vi "Zeiss File Header Tclk.vi"(7 "Write":bool=TRUE, 8 "error in":errorcluster, 9 "Inputs":T2={"AI sampling time increment"=0.0, "8-bit"=TRUE, "AI scaling coefficients"=[], "AI channels"={"AI 1"=FALSE, "AI 2"=FALSE, "AI 3"=FALSE, "AI 4"=FALSE}, "Resolution and scan"={"X resolution"=1, "Z resolution"=1, "AI oversampling"=1, "Scan speed"=1, "Actual AO rate"=1.0, "Frame line rampdown ratio"=1.0, "X min (V)"=0.0, "X max (V)"=0.0, "Det min (V)"=-10.0, "Det max (V)"=10.0}, "Decimating factor"=2, "Notes"="", "Other detectors"={"Detector C name"="", "Detector D name"=""}, "SEM parameters"={"Detector A"="", "Detector B"="Detecter B name", "Brightness A"=0.0, "Contrast A"=0.0, "Brightness B"=0.0, "Contrast B"=0.0, "Magnification"=0.0, "Pixel size"=0.0, "Working distance"=0.0, "EHT"=0.0, "Aperture"=0, "High current mode"=0, "Probe current"=0.0, "Scan rotation"=0.0, "Chamber vac"=0.0, "Gun vac"=0.0, "Beam shift X"=0.0, "Beam shift Y"=0.0, "Stig X"=0.0, "Stig Y"=0.0, "Alignment X"=0.0, "Alignment Y"=0.0, "Stage X"=0.0, "Stage Y"=0.0, "Stage Z"=0.0, "Stage T"=0.0, "Stage R"=0.0, "Stage M"=0.0}, "FIB parameters"={"FIB mode"=0, "FIB focus"=0.0, "FIB probe current"=0, "FIB emission current"=0.0, "FIB rotation"=0.0, "FIB aperture X"=0.0, "FIB aperture Y"=0.0, "FIB stig X"=0.0, "FIB stig Y"=0.0, "FIB beam shift X"=0.0, "FIB beam shift Y"=0.0}, "Milling para"={"X resolution"=4096, "Z resolution"=125001, "X offset (um)"=0.0, "Z offset (um)"=0.0, "X center (um)"=0.0, "Z center (um)"=0.0, "X size (um)"=250.0, "Z size (um)"=250.0, "UL-Ang"=90.0, "UR-Ang"=90.0, "Line milling time (s)"=5.0, "Z-step (nm)"=2.0, "Lines auto pause"=1, "Auto pause"=FALSE, "Mill from Bottom"=FALSE, "FIB FOV (um)"=500.0, "Auto Profile"=FALSE, "Mill start from Last"=FALSE, "FIB PID on"=FALSE, "FIB PID reset"=TRUE, "FIB PID measured"=0, "FIB PID target"=0.0, "FIB PID target slope"=0.0, "FIB PID P"=0.001, "FIB PID I"=0.01, "FIB PID D"=0.0, "Emission (uA)"=1.36, "Suppressor (V)"=50.0, "Auto reheat"=FALSE}, "Machine ID"="", "Data Logging"={"Temp (F)"=0.0, "FIB Faraday Cup (nA)"=0.0, "FIB Specimen I (nA)"=0.0, "Beam Dump 1 (nA)"=0.0, "Beam Dump 2 (nA)"=0.0, "Milling I (nA)"=0.0, "SEM Specimen I (nA)"=0.0, "Milling Z voltage (V)"=0.0, "Focus Index"=0.0, "FIB slice #"=0}} {"Milling para"."Suppressor (V)" step=0.1 format="%.1g"; "Milling para"."Emission (uA)" step=0.1 format="%.2g"; "Milling para"."FIB PID measured" items=["Spec.", "B.D. 1", "B.D. 2", "Mill", "Spec. +"]; "Milling para"."FIB PID target slope" min=-1 max=1 step=0.1; "Milling para"."UR-Ang" format="%.2f"; "Milling para"."UL-Ang" format="%.2f"; "Milling para"."Z offset (um)" step=0.02 format="%.3g"; "Milling para"."X offset (um)" step=1 format="%.3g"; "Milling para"."FIB FOV (um)" format="%.3g"; "Milling para"."Line milling time (s)" format="%.1f"; "Milling para"."Z center (um)" format="%#.3g"; "Milling para"."X center (um)" format="%#.3g"; "Data Logging"."Milling I (nA)" format="%.2g"; "Data Logging"."Beam Dump 2 (nA)" format="%.2g"; "Data Logging"."Focus Index" format="%#_3g"; "Data Logging"."Milling Z voltage (V)" format="%.4g"; "Data Logging"."SEM Specimen I (nA)" format="%.2g"; "Data Logging"."Beam Dump 1 (nA)" format="%.2g"; "Data Logging"."FIB Specimen I (nA)" format="%.2g"; "Data Logging"."FIB Faraday Cup (nA)" format="%.2g"; "Data Logging"."Temp (F)" format="%.2g"}, 10 "Input file path":path, 11 "refnum":refnum<file>) -> (0 "error out":errorcluster, 1 "Ouputs":T1={"AI sampling time increment"=0.0, "AI scaling coefficients"=[], "AI channels"={"AI 1"=FALSE, "AI 2"=FALSE, "AI 3"=FALSE, "AI 4"=FALSE}, "Resolution and scan"={"X resolution"=1, "Z resolution"=1, "AI oversampling"=1, "Scan speed"=1, "Actual AO rate"=1.0, "Frame line rampdown ratio"=1.0, "X min (V)"=0.0, "X max (V)"=0.0, "Det min (V)"=-10.0, "Det max (V)"=10.0}, "Decimating factor"=2, "Notes"="", "Other detectors"={"Detector C name"="", "Detector D name"=""}, "SEM parameters"={"Detector A"="", "Detector B"="Detecter B name", "Brightness A"=0.0, "Contrast A"=0.0, "Brightness B"=0.0, "Contrast B"=0.0, "Magnification"=0.0, "Pixel size"=0.0, "Working distance"=0.0, "EHT"=0.0, "Aperture"=0, "High current mode"=0, "Probe current"=0.0, "Scan rotation"=0.0, "Chamber vac"=0.0, "Gun vac"=0.0, "Beam shift X"=0.0, "Beam shift Y"=0.0, "Stig X"=0.0, "Stig Y"=0.0, "Alignment X"=0.0, "Alignment Y"=0.0, "Stage X"=0.0, "Stage Y"=0.0, "Stage Z"=0.0, "Stage T"=0.0, "Stage R"=0.0, "Stage M"=0.0}, "FIB parameters"={"FIB mode"=0, "FIB focus"=0.0, "FIB probe current"=0, "FIB emission current"=0.0, "FIB rotation"=0.0, "FIB aperture X"=0.0, "FIB aperture Y"=0.0, "FIB stig X"=0.0, "FIB stig Y"=0.0, "FIB beam shift X"=0.0, "FIB beam shift Y"=0.0}, "Milling para"={"X resolution"=4096, "Z resolution"=125001, "X offset (um)"=0.0, "Z offset (um)"=0.0, "X center (um)"=0.0, "Z center (um)"=0.0, "X size (um)"=250.0, "Z size (um)"=250.0, "UL-Ang"=90.0, "UR-Ang"=90.0, "Line milling time (s)"=5.0, "Z-step (nm)"=2.0, "Lines auto pause"=1, "Auto pause"=FALSE, "Mill from Bottom"=FALSE, "FIB FOV (um)"=500.0, "Auto Profile"=FALSE, "Mill start from Last"=FALSE, "FIB PID on"=FALSE, "FIB PID reset"=TRUE, "FIB PID measured"=0, "FIB PID target"=0.0, "FIB PID target slope"=0.0, "FIB PID P"=0.001, "FIB PID I"=0.01, "FIB PID D"=0.0, "Emission (uA)"=1.36, "Suppressor (V)"=50.0, "Auto reheat"=FALSE}, "Machine ID"="", "Data Logging"={"Temp (F)"=0.0, "FIB Faraday Cup (nA)"=0.0, "FIB Specimen I (nA)"=0.0, "Beam Dump 1 (nA)"=0.0, "Beam Dump 2 (nA)"=0.0, "Milling I (nA)"=0.0, "SEM Specimen I (nA)"=0.0, "Milling Z voltage (V)"=0.0, "Focus Index"=0.0, "FIB slice #"=0}} {"Milling para"."Suppressor (V)" step=0.1 format="%.1g"; "Milling para"."Emission (uA)" step=0.1 format="%.2g"; "Milling para"."FIB PID measured" items=["Spec.", "B.D. 1", "B.D. 2", "Mill", "Spec. +"]; "Milling para"."FIB PID target slope" min=-1 max=1 step=0.1; "Milling para"."UR-Ang" format="%.2f"; "Milling para"."UL-Ang" format="%.2f"; "Milling para"."Z offset (um)" step=0.02 format="%.3g"; "Milling para"."X offset (um)" step=1 format="%.3g"; "Milling para"."FIB FOV (um)" format="%.3g"; "Milling para"."Line milling time (s)" format="%.1f"; "Milling para"."Z center (um)" format="%#.3g"; "Milling para"."X center (um)" format="%#.3g"; "Data Logging"."Milling I (nA)" format="%.2g"; "Data Logging"."Beam Dump 2 (nA)" format="%.2g"; "Data Logging"."Focus Index" format="%#_3g"; "Data Logging"."Milling Z voltage (V)" format="%.4g"; "Data Logging"."SEM Specimen I (nA)" format="%.2g"; "Data Logging"."Beam Dump 1 (nA)" format="%.2g"; "Data Logging"."FIB Specimen I (nA)" format="%.2g"; "Data Logging"."FIB Faraday Cup (nA)" format="%.2g"; "Data Logging"."Temp (F)" format="%.2g"}, 3 "dup refnum":refnum<file>)   [LabVIEW 2018]
panel:
  in  "Detector calibration":sgl[](array[numeric])=[0.0, 0.0, 0.0, 0.0]
  out "SW date":string
  out "Detectors":refnum<k15>="PXI1Slot3"
  # "Direction"
  # "Start\nfrom"
  # "<"
  # "Direction"
  # "Start\nfrom"
  # "<"
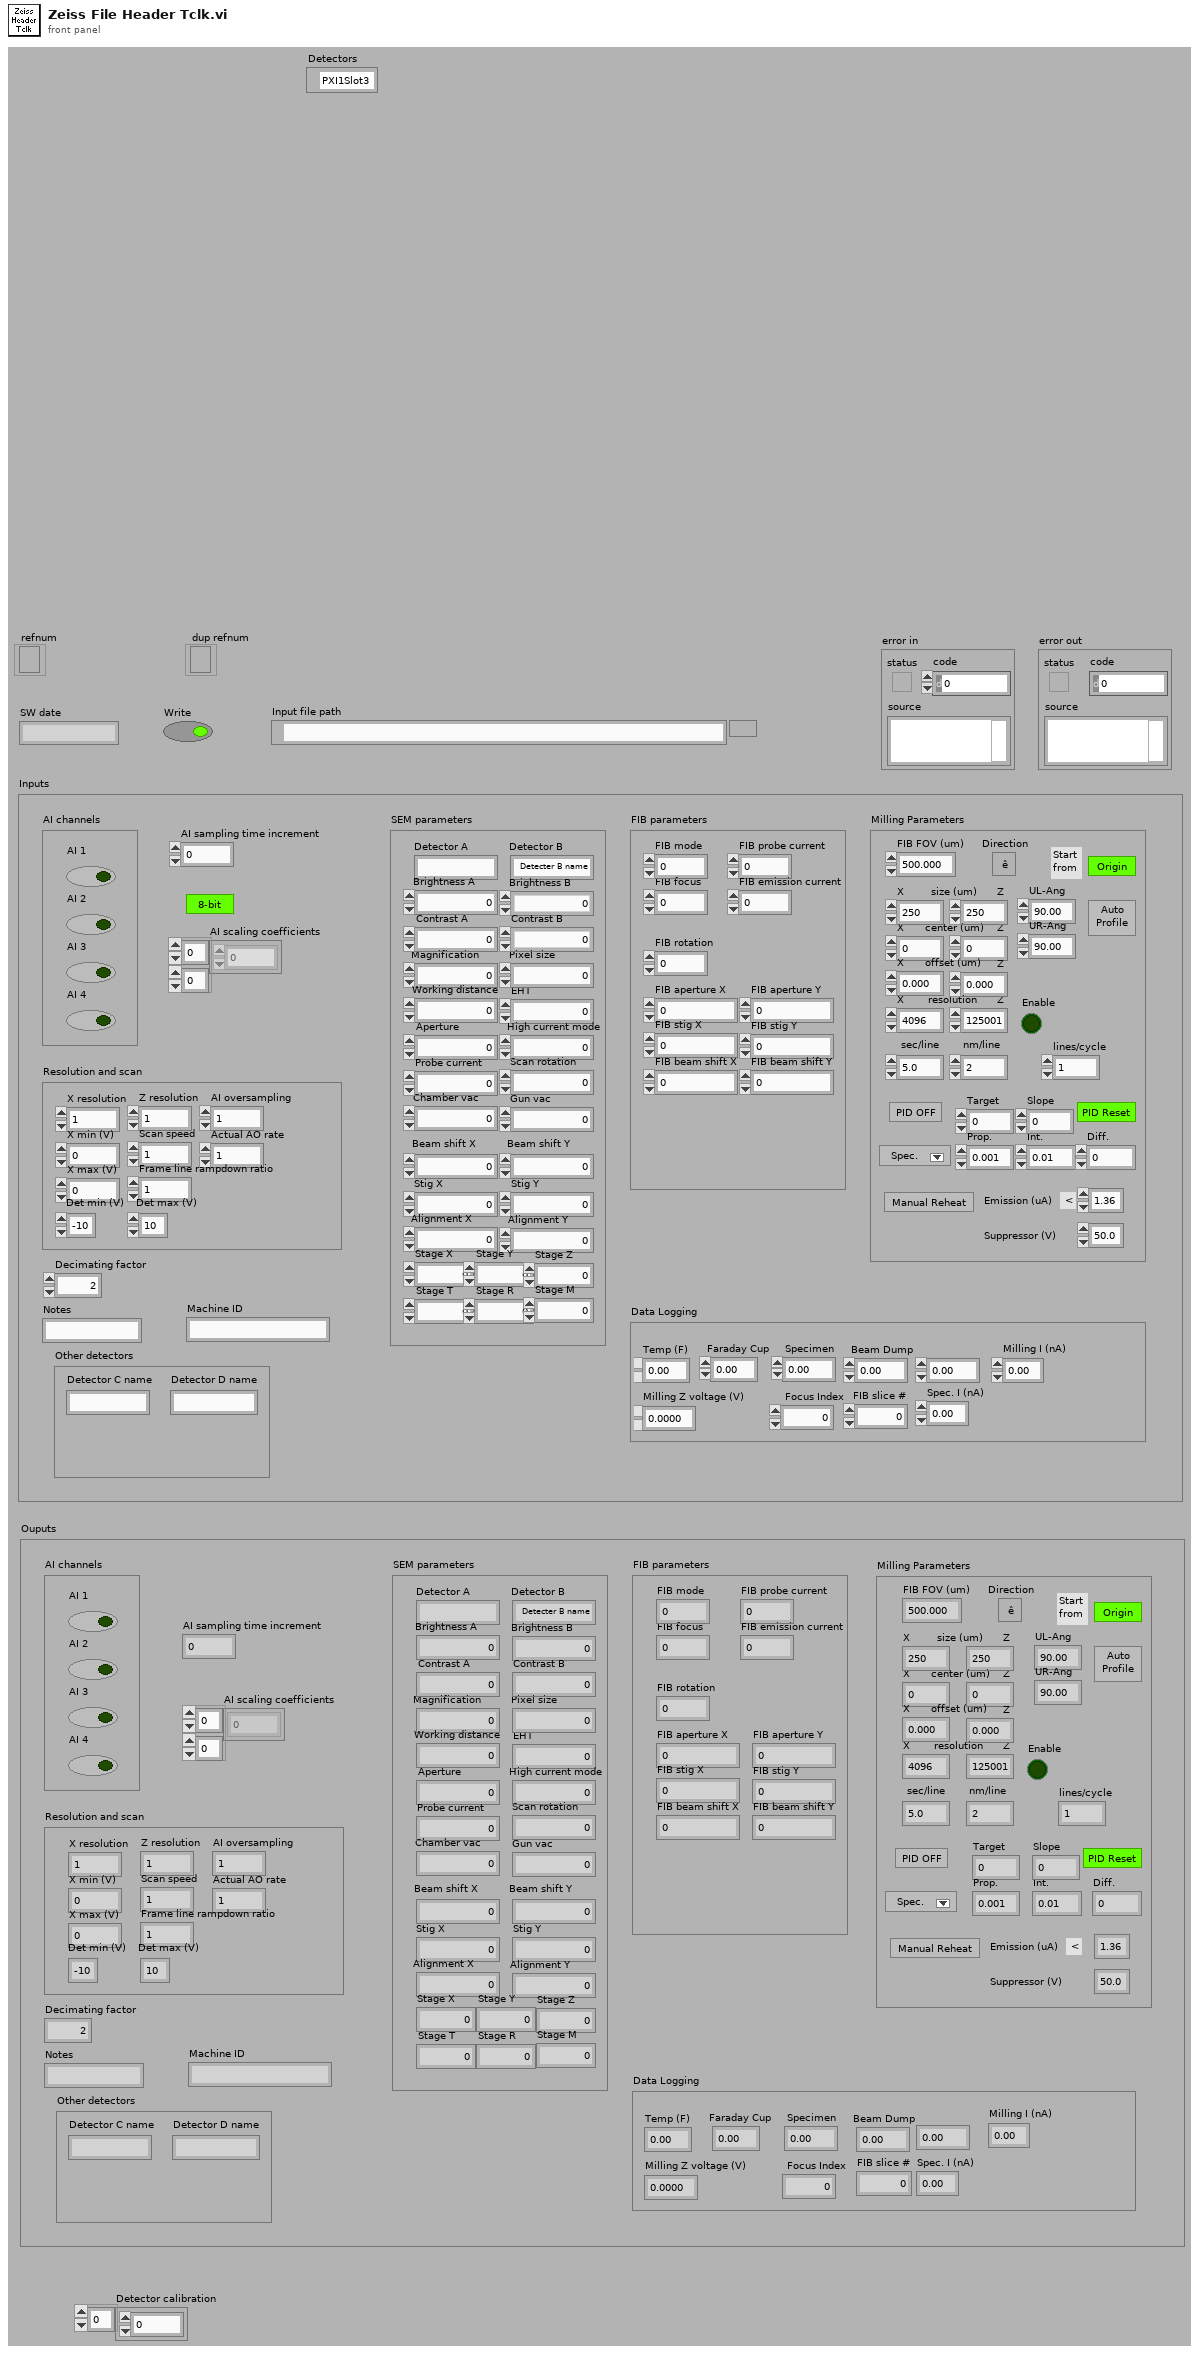
[diagram p1: front panel]
types:
  T1 = cluster{"AI sampling time increment":dbl, "AI scaling coefficients":sgl[][], "AI channels":cluster{"AI 1":bool, "AI 2":bool, "AI 3":bool, "AI 4":bool}, "Resolution and scan":cluster{"X resolution":u32, "Z resolution":u32, "AI oversampling":u16, "Scan speed":u8, "Actual AO rate":dbl, "Frame line rampdown ratio":dbl, "X min (V)":dbl, "X max (V)":dbl, "Det min (V)":dbl, "Det max (V)":dbl}, "Decimating factor":u16, "Notes":string, "Other detectors":cluster{"Detector C name":string, "Detector D name":string}, "SEM parameters":cluster{"Detector A":string, "Detector B":string, "Brightness A":sgl, "Contrast A":sgl, "Brightness B":sgl, "Contrast B":sgl, "Magnification":sgl, "Pixel size":sgl, "Working distance":sgl, "EHT":sgl, "Aperture":u8, "High current mode":u8, "Probe current":sgl, "Scan rotation":sgl, "Chamber vac":sgl, "Gun vac":sgl, "Beam shift X":sgl, "Beam shift Y":sgl, "Stig X":sgl, "Stig Y":sgl, "Alignment X":sgl, "Alignment Y":sgl, "Stage X":sgl, "Stage Y":sgl, "Stage Z":sgl, "Stage T":sgl, "Stage R":sgl, "Stage M":sgl}, "FIB parameters":cluster{"FIB mode":u8, "FIB focus":sgl, "FIB probe current":u8, "FIB emission current":sgl, "FIB rotation":sgl, "FIB aperture X":sgl, "FIB aperture Y":sgl, "FIB stig X":sgl, "FIB stig Y":sgl, "FIB beam shift X":sgl, "FIB beam shift Y":sgl}, "Milling para":cluster{"X resolution":u32, "Z resolution":u32, "X offset (um)":sgl, "Z offset (um)":sgl, "X center (um)":sgl, "Z center (um)":sgl, "X size (um)":sgl, "Z size (um)":sgl, "UL-Ang":sgl, "UR-Ang":sgl, "Line milling time (s)":sgl, "Z-step (nm)":dbl, "Lines auto pause":u16, "Auto pause":bool, "Mill from Bottom":bool, "FIB FOV (um)":sgl, "Auto Profile":bool, "Mill start from Last":bool, "FIB PID on":bool, "FIB PID reset":bool, "FIB PID measured":u8, "FIB PID target":sgl, "FIB PID target slope":sgl, "FIB PID P":sgl, "FIB PID I":sgl, "FIB PID D":sgl, "Emission (uA)":dbl, "Suppressor (V)":sgl, "Auto reheat":bool}, "Machine ID":string, "Data Logging":cluster{"Temp (F)":sgl, "FIB Faraday Cup (nA)":sgl, "FIB Specimen I (nA)":sgl, "Beam Dump 1 (nA)":sgl, "Beam Dump 2 (nA)":sgl, "Milling I (nA)":sgl, "SEM Specimen I (nA)":sgl, "Milling Z voltage (V)":sgl, "Focus Index":sgl, "FIB slice #":u32}}
  T2 = cluster{"AI sampling time increment":dbl, "8-bit":bool, "AI scaling coefficients":sgl[][], "AI channels":cluster{"AI 1":bool, "AI 2":bool, "AI 3":bool, "AI 4":bool}, "Resolution and scan":cluster{"X resolution":u32, "Z resolution":u32, "AI oversampling":u16, "Scan speed":u8, "Actual AO rate":dbl, "Frame line rampdown ratio":dbl, "X min (V)":dbl, "X max (V)":dbl, "Det min (V)":dbl, "Det max (V)":dbl}, "Decimating factor":u16, "Notes":string, "Other detectors":cluster{"Detector C name":string, "Detector D name":string}, "SEM parameters":cluster{"Detector A":string, "Detector B":string, "Brightness A":sgl, "Contrast A":sgl, "Brightness B":sgl, "Contrast B":sgl, "Magnification":sgl, "Pixel size":sgl, "Working distance":sgl, "EHT":sgl, "Aperture":u8, "High current mode":u8, "Probe current":sgl, "Scan rotation":sgl, "Chamber vac":sgl, "Gun vac":sgl, "Beam shift X":sgl, "Beam shift Y":sgl, "Stig X":sgl, "Stig Y":sgl, "Alignment X":sgl, "Alignment Y":sgl, "Stage X":sgl, "Stage Y":sgl, "Stage Z":sgl, "Stage T":sgl, "Stage R":sgl, "Stage M":sgl}, "FIB parameters":cluster{"FIB mode":u8, "FIB focus":sgl, "FIB probe current":u8, "FIB emission current":sgl, "FIB rotation":sgl, "FIB aperture X":sgl, "FIB aperture Y":sgl, "FIB stig X":sgl, "FIB stig Y":sgl, "FIB beam shift X":sgl, "FIB beam shift Y":sgl}, "Milling para":cluster{"X resolution":u32, "Z resolution":u32, "X offset (um)":sgl, "Z offset (um)":sgl, "X center (um)":sgl, "Z center (um)":sgl, "X size (um)":sgl, "Z size (um)":sgl, "UL-Ang":sgl, "UR-Ang":sgl, "Line milling time (s)":sgl, "Z-step (nm)":dbl, "Lines auto pause":u16, "Auto pause":bool, "Mill from Bottom":bool, "FIB FOV (um)":sgl, "Auto Profile":bool, "Mill start from Last":bool, "FIB PID on":bool, "FIB PID reset":bool, "FIB PID measured":u8, "FIB PID target":sgl, "FIB PID target slope":sgl, "FIB PID P":sgl, "FIB PID I":sgl, "FIB PID D":sgl, "Emission (uA)":dbl, "Suppressor (V)":sgl, "Auto reheat":bool}, "Machine ID":string, "Data Logging":cluster{"Temp (F)":sgl, "FIB Faraday Cup (nA)":sgl, "FIB Specimen I (nA)":sgl, "Beam Dump 1 (nA)":sgl, "Beam Dump 2 (nA)":sgl, "Milling I (nA)":sgl, "SEM Specimen I (nA)":sgl, "Milling Z voltage (V)":sgl, "Focus Index":sgl, "FIB slice #":u32}}
  T3 = cluster{"Detector C name":string, "Detector D name":string}
  T4 = cluster{"FIB mode":u8, "FIB focus":sgl, "FIB probe current":u8, "FIB emission current":sgl, "FIB rotation":sgl, "FIB aperture X":sgl, "FIB aperture Y":sgl, "FIB stig X":sgl, "FIB stig Y":sgl, "FIB beam shift X":sgl, "FIB beam shift Y":sgl}
  T5 = cluster{"Temp (F)":sgl, "FIB Faraday Cup (nA)":sgl, "FIB Specimen I (nA)":sgl, "Beam Dump 1 (nA)":sgl, "Beam Dump 2 (nA)":sgl, "Milling I (nA)":sgl, "SEM Specimen I (nA)":sgl, "Milling Z voltage (V)":sgl, "Focus Index":sgl, "FIB slice #":u32}
  T6 = cluster{"Detector A":string, "Detector B":string, "Brightness A":sgl, "Contrast A":sgl, "Brightness B":sgl, "Contrast B":sgl, "Magnification":sgl, "Pixel size":sgl, "Working distance":sgl, "EHT":sgl, "Aperture":u8, "High current mode":u8, "Probe current":sgl, "Scan rotation":sgl, "Chamber vac":sgl, "Gun vac":sgl, "Beam shift X":sgl, "Beam shift Y":sgl, "Stig X":sgl, "Stig Y":sgl, "Alignment X":sgl, "Alignment Y":sgl, "Stage X":sgl, "Stage Y":sgl, "Stage Z":sgl, "Stage T":sgl, "Stage R":sgl, "Stage M":sgl}
  T7 = cluster{"AI 1":bool, "AI 2":bool, "AI 3":bool, "AI 4":bool}
  T8 = cluster{"X resolution":u32, "Z resolution":u32, "AI oversampling":u16, "Scan speed":u8, "Actual AO rate":dbl, "Frame line rampdown ratio":dbl, "X min (V)":dbl, "X max (V)":dbl, "Det min (V)":dbl, "Det max (V)":dbl}
  T9 = cluster{"X resolution":u32, "Z resolution":u32, "X offset (um)":sgl, "Z offset (um)":sgl, "X center (um)":sgl, "Z center (um)":sgl, "X size (um)":sgl, "Z size (um)":sgl, "UL-Ang":sgl, "UR-Ang":sgl, "Line milling time (s)":sgl, "Z-step (nm)":dbl, "Lines auto pause":u16, "Auto pause":bool, "Mill from Bottom":bool, "FIB FOV (um)":sgl, "Auto Profile":bool, "Mill start from Last":bool, "FIB PID on":bool, "FIB PID reset":bool, "FIB PID measured":u8, "FIB PID target":sgl, "FIB PID target slope":sgl, "FIB PID P":sgl, "FIB PID I":sgl, "FIB PID D":sgl, "Emission (uA)":dbl, "Suppressor (V)":sgl, "Auto reheat":bool}
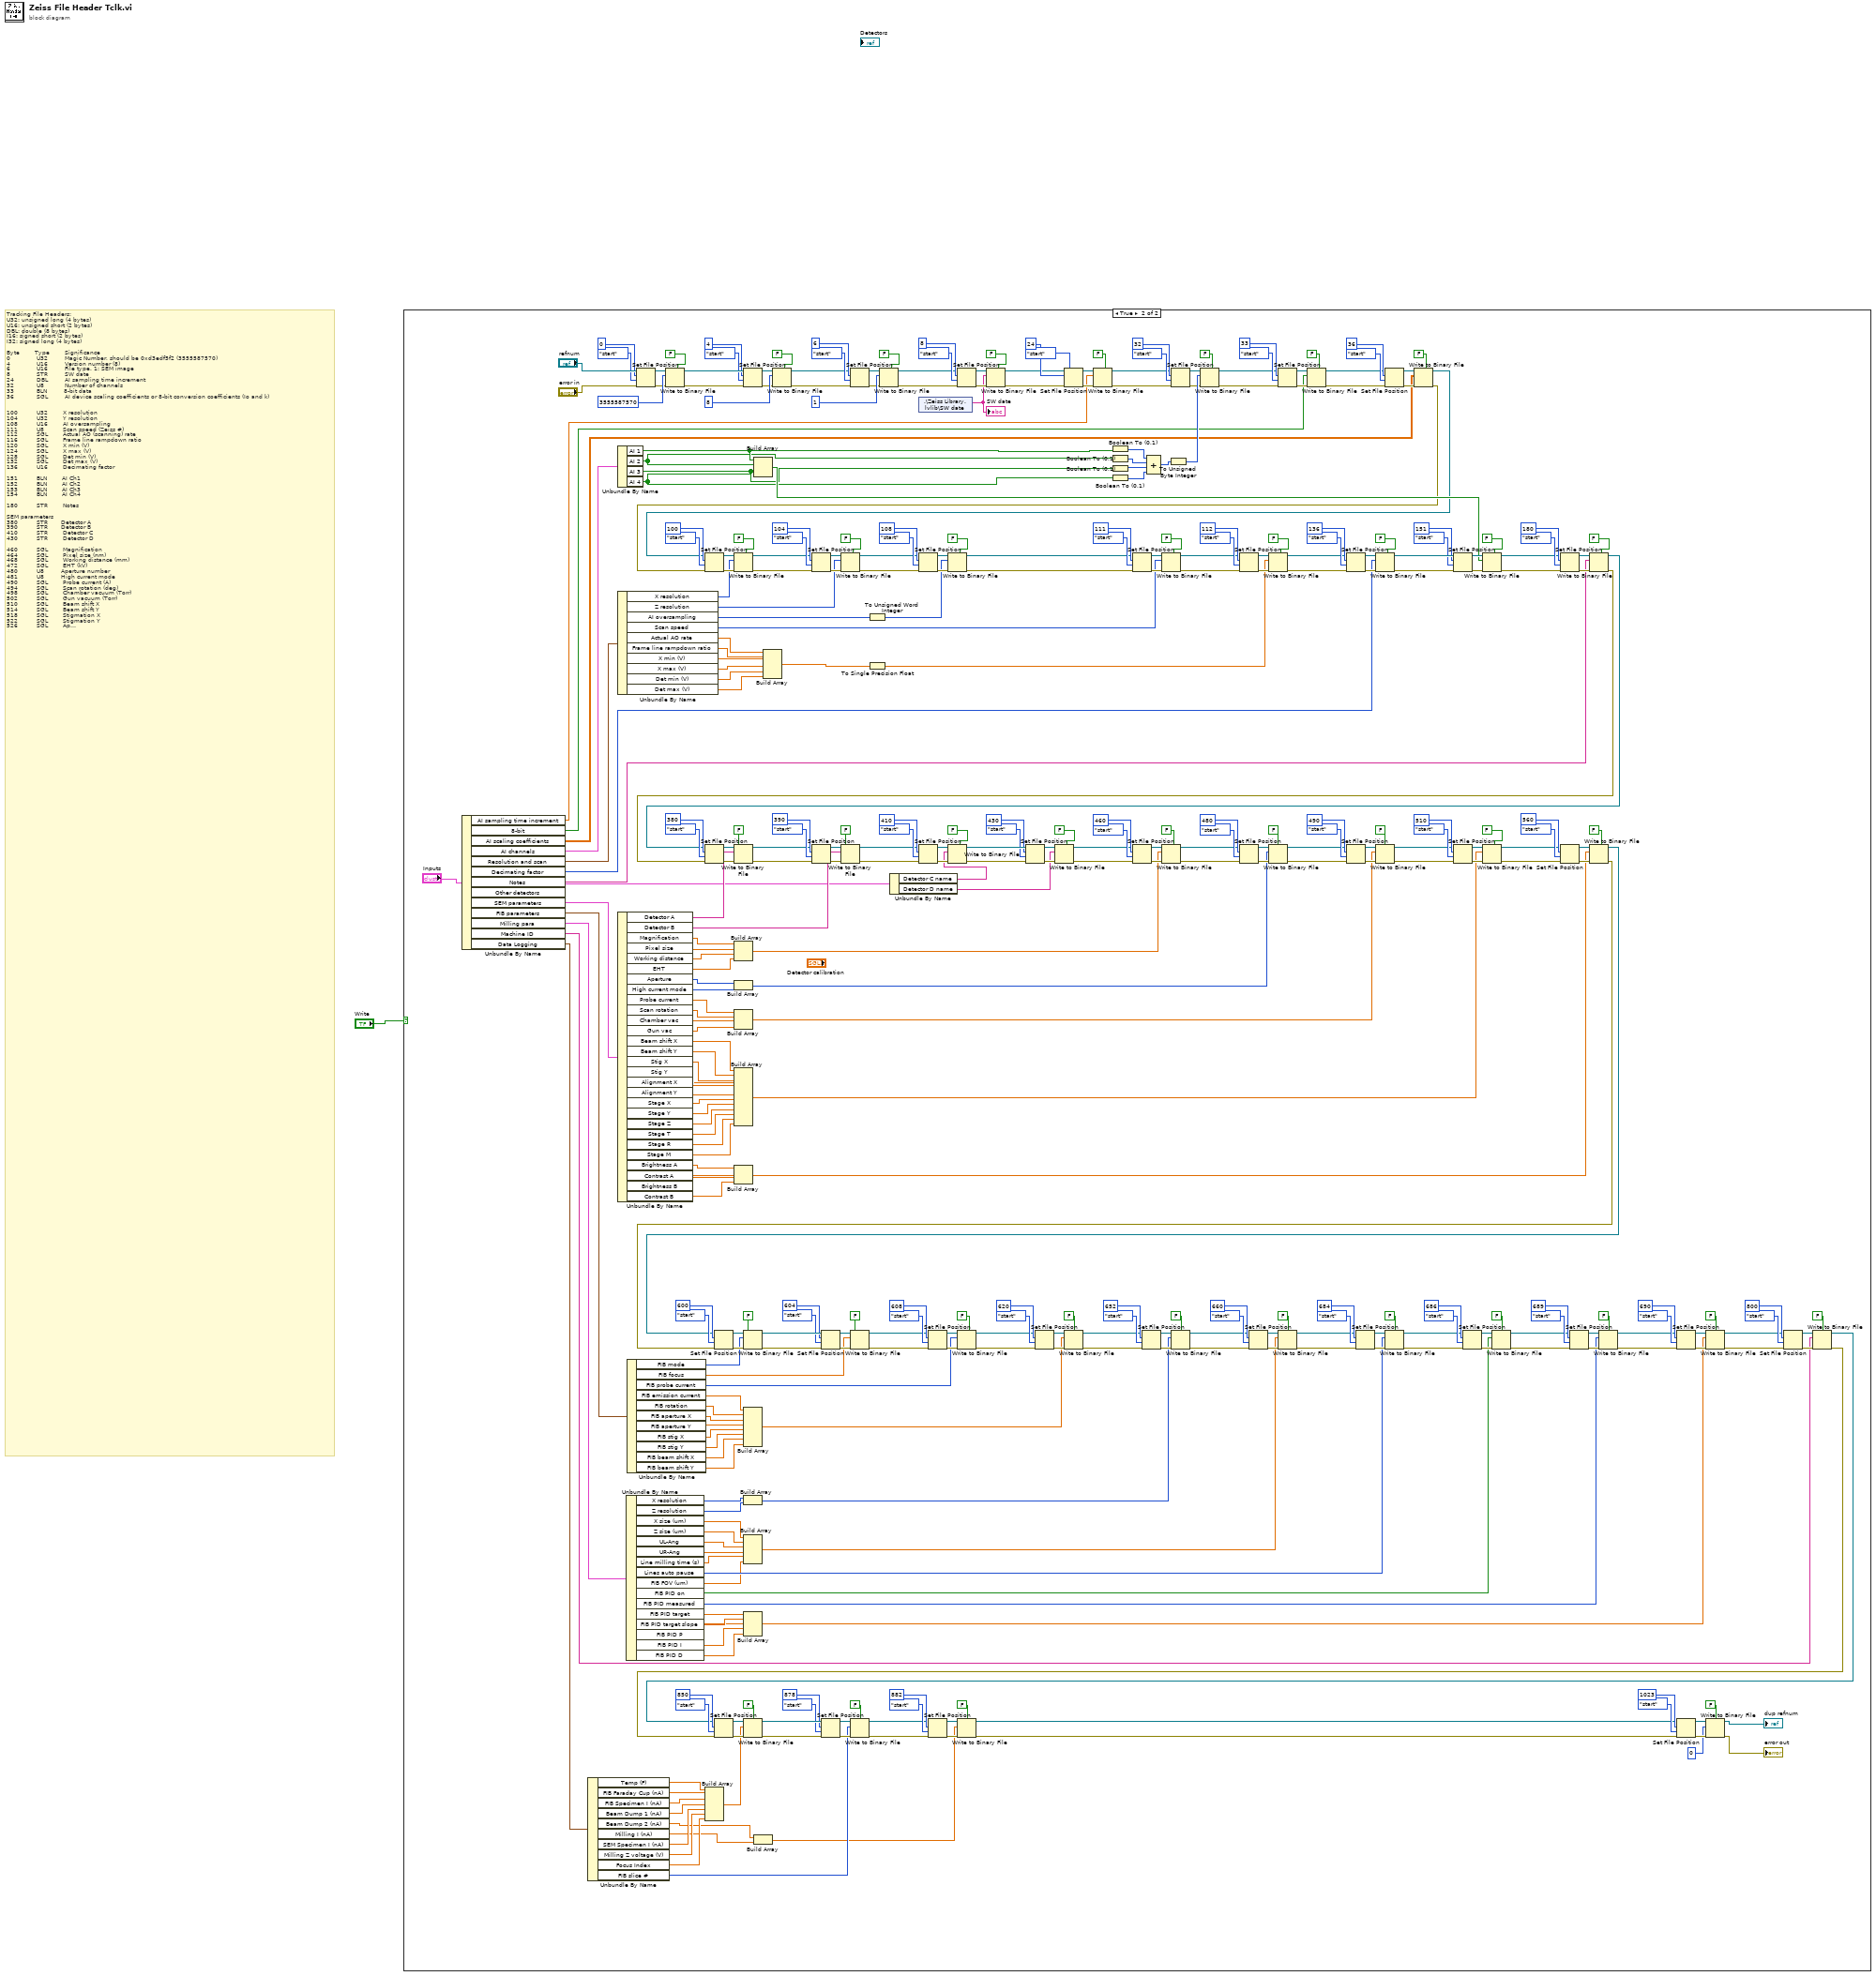
[diagram p0: block diagram]
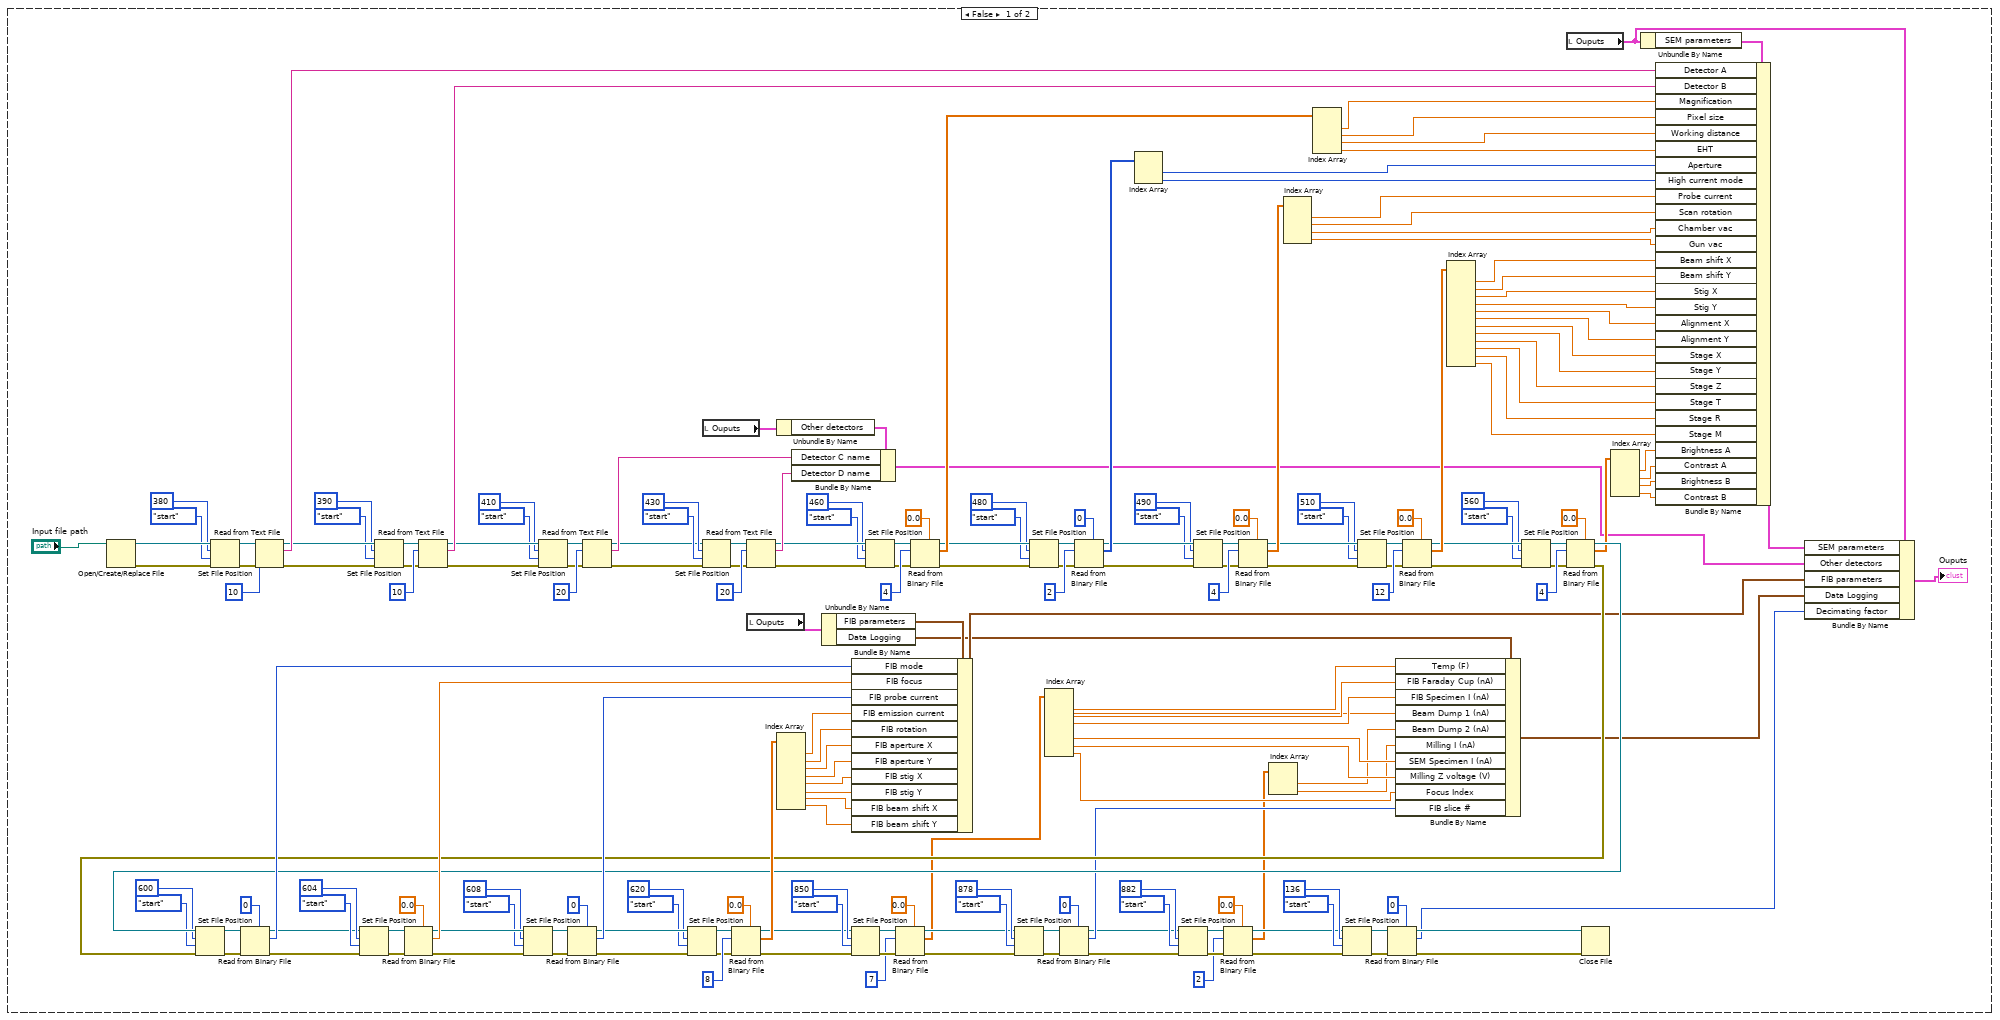
[diagram p2: hidden frame]
diagram:
  # "Tracking File Headers:\nU32: unsigned long (4 bytes)\nU16: unsigned short (2 bytes)\nDBL: double (8 bytes)\nI16: signed short (2 bytes)\nI32: signed long (4 bytes)\n\nByte\t       Type\t\t      Significance\n0              U32\t        Magic Number, should be 0xd3edf5f2 (3555587570)\n4   \t          U16\t        Version number (8)\n6   \t          U16\t        File type. 1: SEM image\n8              STR         SW date\n24     \t      DBL         AI sampling time increment\n32     \t      U8           Number of channels\n33            BLN         8-bit data\n36            SGL         AI device scaling coefficients or 8-bit conversion coefficients (Io and k)\n\n\n100          U32        X resolution\n104          U32        Y resolution\n108          U16        AI oversampling     \n111          U8          Scan speed (Zeiss #)\n112          SGL        Actual AO (scanning) rate\n116          SGL        Frame line rampdown ratio\n120          SGL        X min (V)\n124          SGL        X max (V)\n128          SGL        Det min (V)\n132          SGL        Det max (V)\n136          U16        Decimating factor \n\n151          BLN        AI Ch1          \n152          BLN        AI Ch2\n153          BLN        AI Ch3\n154          BLN        AI Ch4\n \n180          STR        Notes\n\nSEM parameters\n380          STR       Detector A\n390          STR       Detector B\n410          STR        Detector C\n430          STR        Detector D\n\n460          SGL        Magnification\n464          SGL        Pixel size (nm)\n468          SGL        Working distance (mm)\n472          SGL        EHT (kV)\n480          U8         Aperture number\n481          U8         High current mode\n490          SGL        Probe current (A)\n494          SGL        Scan rotation (deg)\n498          SGL        Chamber vacuum (Torr)\n502          SGL        Gun vacuum (Torr)\n510          SGL        Beam shift X\n514          SGL        Beam shift Y\n518          SGL        Stigmation X\n522          SGL        Stigmation Y\n526          SGL        Aperture aligment X\n530          SGL        Aperture aligment Y\n534          SGL        Stage X (mm)\n538          SGL        Stage Y (mm)\n542          SGL        Stage Z (mm)\n546          SGL        Stage T (deg)\n550          SGL        Stage R (deg)\n554          SGL        Stage M (mm)\n560          SGL        Brightness (%), detector A\n564          SGL        Contrast (%),  detector A\n568          SGL        Brightness (%), detector B\n572          SGL        Contrast (%),  detector B\n\n\nFIB parameters\n600          U8         Mode\n604          SGL        Focus (V)\n608          U8         Probe current number\n620          SGL        Emission current (A)\n624          SGL        rotation (deg)\n628          SGL        Aperture alignment X\n632          SGL        Aperture alignment Y\n636          SGL        Stigmation X\n640          SGL        Stigmation Y\n644          SGL        Beam shift X (um)\n648          SGL        Beam shift Y (um)\n\n\nMilling parameters\n652          U32        X resolution\n656          U32        Y resolution\n660          SGL        X size (um)\n664          SGL        Y size (um)\n668          SGL        UL-Ang (deg)\n672          SGL        UR-Ang (deg)\n676          SGL        Line milling time (s)\n680          SGL        FIB FOV (um)\n684          U16        Lines auto pause\n686          BLN       FIB PID on\n689          U8          FIB PID measured (0: specimen, 1: beam dump)\n690          SGL        FIB PID target\n694          SGL        FIB PID target slope\n698          SGL        FIB PID P\n702          SGL        FIB PID I\n706          SGL        FIB PID D\n\n\n800          STR        Machine ID\n\n850          SGL        Temperature (F)\n854          SGL        Faraday cup current (nA)\n858          SGL        Specimen current during FIB (nA)\n862          SGL        Beam dump 1 current (nA)\n866          SGL        Specimen current during SEM (nA)\n870          SGL        Milling Z voltage (V)\n874          SGL        Focus index\n878          U32        FIB slice #\n882          SGL        Beam dump 2 current (nA)\n886          SGL        Milling current (nA)\n\n1000        DBL        File length, position for the beginning of recipe variant\n\n1024        I16          1-D array of n channels of unscaled measurement from DAQ"
  n1 = case shown="True" "Write" {
    frame False {
      n2 = Open/Create/Replace File(file path (use dialog)="Input file path") -> (refnum out=w111:refnum<file>, error out=w112:errorcluster)  [unwired: 5 in, 1 out]
      n3 = Set File Position(offset (in bytes) (0)=380 ("pos offset (0)"), refnum=w111, from (0:start)=enum16{"start", "end", "current"}."start" ("pos mode (0:2)"), error in=w112) -> (refnum out=w81:refnum<file>, error out=w82:errorcluster)
      n4 = Read from Text File(file (use dialog)=w81, count=10, error in=w82) -> (refnum out=w91:refnum<file>, text=w121:string, error out=w92:errorcluster)  [unwired: 1 in, 1 out]
      n5 = Set File Position(offset (in bytes) (0)=390 ("pos offset (0)"), refnum=w91, from (0:start)=enum16{"start", "end", "current"}."start" ("pos mode (0:2)"), error in=w92) -> (refnum out=w89:refnum<file>, error out=w90:errorcluster)
      n6 = Read from Text File(file (use dialog)=w89, count=10, error in=w90) -> (refnum out=w103:refnum<file>, text=w122:string, error out=w104:errorcluster)  [unwired: 1 in, 1 out]
      n7 = Set File Position(offset (in bytes) (0)=410 ("pos offset (0)"), refnum=w103, from (0:start)=enum16{"start", "end", "current"}."start" ("pos mode (0:2)"), error in=w104) -> (refnum out=w96:refnum<file>, error out=w95:errorcluster)
      n8 = Read from Text File(file (use dialog)=w96, count=20, error in=w95) -> (refnum out=w94:refnum<file>, text=w119:string, error out=w93:errorcluster)  [unwired: 1 in, 1 out]
      n9 = local read "Ouputs"() -> (w57:T1)
      n10 = Set File Position(offset (in bytes) (0)=430 ("pos offset (0)"), refnum=w94, from (0:start)=enum16{"start", "end", "current"}."start" ("pos mode (0:2)"), error in=w93) -> (refnum out=w101:refnum<file>, error out=w102:errorcluster)
      n11 = Read from Text File(file (use dialog)=w101, count=20, error in=w102) -> (refnum out=w105:refnum<file>, text=w120:string, error out=w106:errorcluster)  [unwired: 1 in, 1 out]
      n12 = local read "Ouputs"() -> (w55:T1)
      n13 = Unbundle By Name(w57) -> ("Other detectors"=w56:T3)
      n14 = Bundle By Name(cluster=w56, "Detector C name"=w119, "Detector D name"=w120) -> (w50:T3)
      n15 = Unbundle By Name(w55) -> ("FIB parameters"=w54:T4, "Data Logging"=w24:T5)
      n16 = Set File Position(offset (in bytes) (0)=460 ("pos offset (0)"), refnum=w105, from (0:start)=enum16{"start", "end", "current"}."start" ("pos mode (0:2)"), error in=w106) -> (refnum out=w79:refnum<file>, error out=w80:errorcluster)
      n17 = Read from Binary File(5:sgl 0.0, 8:w80, 10:4 ("count (1)"), 11:w79) -> (0:w70:errorcluster, 2:w124:sgl[], 3:w69:refnum<file>)  [unwired: 2 in, 1 out]
      n18 = Set File Position(offset (in bytes) (0)=480 ("pos offset (0)"), refnum=w69, from (0:start)=enum16{"start", "end", "current"}."start" ("pos mode (0:2)"), error in=w70) -> (refnum out=w77:refnum<file>, error out=w78:errorcluster)
      n19 = Read from Binary File(5:u8 0, 8:w78, 10:2 ("count (1)"), 11:w77) -> (0:w74:errorcluster, 2:w130:u8[], 3:w73:refnum<file>)  [unwired: 2 in, 1 out]
      n20 = Index Array(array=w130) -> (element #1=w131:u8, element #2=w132:u8)  [unwired: 2 in]
      n21 = Set File Position(offset (in bytes) (0)=490 ("pos offset (0)"), refnum=w73, from (0:start)=enum16{"start", "end", "current"}."start" ("pos mode (0:2)"), error in=w74) -> (refnum out=w75:refnum<file>, error out=w76:errorcluster)
      n22 = Read from Binary File(5:sgl 0.0, 8:w76, 10:4 ("count (1)"), 11:w75) -> (0:w110:errorcluster, 2:w134:sgl[], 3:w109:refnum<file>)  [unwired: 2 in, 1 out]
      n23 = Index Array(array=w134) -> (element #1=w137:sgl, element #2=w138:sgl, element #3=w139:sgl, element #4=w140:sgl)  [unwired: 4 in]
      n24 = Index Array(array=w124) -> (element #1=w125:sgl, element #2=w126:sgl, element #3=w128:sgl, element #4=w127:sgl)  [unwired: 4 in]
      n25 = Set File Position(offset (in bytes) (0)=510 ("pos offset (0)"), refnum=w109, from (0:start)=enum16{"start", "end", "current"}."start" ("pos mode (0:2)"), error in=w110) -> (refnum out=w84:refnum<file>, error out=w83:errorcluster)
      n26 = Read from Binary File(5:sgl 0.0, 8:w83, 10:12 ("count (1)"), 11:w84) -> (0:w108:errorcluster, 2:w142:sgl[], 3:w107:refnum<file>)  [unwired: 2 in, 1 out]
      n27 = Index Array(array=w142) -> (element #1=w141:sgl, element #2=w143:sgl, element #3=w144:sgl, element #4=w145:sgl, element #5=w146:sgl, element #6=w147:sgl, element #7=w148:sgl, element #8=w149:sgl, element #9=w150:sgl, element #10=w151:sgl, element #11=w152:sgl, element #12=w153:sgl)  [unwired: 12 in]
      n28 = Set File Position(offset (in bytes) (0)=560 ("pos offset (0)"), refnum=w107, from (0:start)=enum16{"start", "end", "current"}."start" ("pos mode (0:2)"), error in=w108) -> (refnum out=w60:refnum<file>, error out=w59:errorcluster)
      n29 = local read "Ouputs"() -> (w52:T1)
      n30 = Read from Binary File(5:sgl 0.0, 8:w59, 10:4 ("count (1)"), 11:w60) -> (0:w182:errorcluster, 2:w155:sgl[], 3:w181:refnum<file>)  [unwired: 2 in, 1 out]
      n31 = Set File Position(offset (in bytes) (0)=600 ("pos offset (0)"), refnum=w181, from (0:start)=enum16{"start", "end", "current"}."start" ("pos mode (0:2)"), error in=w182) -> (refnum out=w160:refnum<file>, error out=w159:errorcluster)
      n32 = Read from Binary File(5:u8 0, 8:w159, 11:w160) -> (0:w164:errorcluster, 2:w188:u8, 3:w163:refnum<file>)  [unwired: 3 in, 1 out]
      n33 = Set File Position(offset (in bytes) (0)=604 ("pos offset (0)"), refnum=w163, from (0:start)=enum16{"start", "end", "current"}."start" ("pos mode (0:2)"), error in=w164) -> (refnum out=w179:refnum<file>, error out=w180:errorcluster)
      n34 = Read from Binary File(5:sgl 0.0, 8:w180, 11:w179) -> (0:w170:errorcluster, 2:w189:sgl, 3:w169:refnum<file>)  [unwired: 3 in, 1 out]
      n35 = Set File Position(offset (in bytes) (0)=608 ("pos offset (0)"), refnum=w169, from (0:start)=enum16{"start", "end", "current"}."start" ("pos mode (0:2)"), error in=w170) -> (refnum out=w177:refnum<file>, error out=w178:errorcluster)
      n36 = Read from Binary File(5:u8 0, 8:w178, 11:w177) -> (0:w174:errorcluster, 2:w190:u8, 3:w173:refnum<file>)  [unwired: 3 in, 1 out]
      n37 = Set File Position(offset (in bytes) (0)=620 ("pos offset (0)"), refnum=w173, from (0:start)=enum16{"start", "end", "current"}."start" ("pos mode (0:2)"), error in=w174) -> (refnum out=w175:refnum<file>, error out=w176:errorcluster)
      n38 = Read from Binary File(5:sgl 0.0, 8:w176, 10:8 ("count (1)"), 11:w175) -> (0:w36:errorcluster, 2:w191:sgl[], 3:w37:refnum<file>)  [unwired: 2 in, 1 out]
      n39 = Index Array(array=w191) -> (element #1=w192:sgl, element #2=w193:sgl, element #3=w194:sgl, element #4=w195:sgl, element #5=w196:sgl, element #6=w197:sgl, element #7=w198:sgl, element #8=w199:sgl)  [unwired: 8 in]
      n40 = Bundle By Name(cluster=w54, "FIB mode"=w188, "FIB focus"=w189, "FIB probe current"=w190, "FIB emission current"=w192, "FIB rotation"=w193, "FIB aperture X"=w194, "FIB aperture Y"=w195, "FIB stig X"=w196, "FIB stig Y"=w197, "FIB beam shift X"=w198, "FIB beam shift Y"=w199) -> (w49:T4)
      n41 = Set File Position(offset (in bytes) (0)=850 ("pos offset (0)"), refnum=w37, from (0:start)=enum16{"start", "end", "current"}."start" ("pos mode (0:2)"), error in=w36) -> (refnum out=w46:refnum<file>, error out=w45:errorcluster)
      n42 = Read from Binary File(5:sgl 0.0, 8:w45, 10:7 ("count (1)"), 11:w46) -> (0:w34:errorcluster, 2:w33:sgl[], 3:w35:refnum<file>)  [unwired: 2 in, 1 out]
      n43 = Set File Position(offset (in bytes) (0)=878 ("pos offset (0)"), refnum=w35, from (0:start)=enum16{"start", "end", "current"}."start" ("pos mode (0:2)"), error in=w34) -> (refnum out=w40:refnum<file>, error out=w41:errorcluster)
      n44 = Index Array(array=w33) -> (element #1=w32:sgl, element #2=w31:sgl, element #3=w30:sgl, element #4=w29:sgl, element #5=w28:sgl, element #6=w27:sgl, element #7=w26:sgl)  [unwired: 7 in]
      n45 = Read from Binary File(5:u32 0, 8:w41, 11:w40) -> (0:w8:errorcluster, 2:w25:u32, 3:w9:refnum<file>)  [unwired: 3 in, 1 out]
      n46 = Set File Position(offset (in bytes) (0)=882 ("pos offset (0)"), refnum=w9, from (0:start)=enum16{"start", "end", "current"}."start" ("pos mode (0:2)"), error in=w8) -> (refnum out=w12:refnum<file>, error out=w13:errorcluster)
      n47 = Read from Binary File(5:sgl 0.0, 8:w13, 10:2 ("count (1)"), 11:w12) -> (0:w6:errorcluster, 2:w5:sgl[], 3:w7:refnum<file>)  [unwired: 2 in, 1 out]
      n48 = Index Array(array=w5) -> (element #1=w3:sgl, element #2=w2:sgl)  [unwired: 2 in]
      n49 = Set File Position(offset (in bytes) (0)=136 ("pos offset (0)"), refnum=w7, from (0:start)=enum16{"start", "end", "current"}."start" ("pos mode (0:2)"), error in=w6) -> (refnum out=w20:refnum<file>, error out=w19:errorcluster)
      n50 = Read from Binary File(5:u16 0, 8:w19, 11:w20) -> (0:w16:errorcluster, 2:w15:u16, 3:w17:refnum<file>)  [unwired: 3 in, 1 out]
      n51 = Bundle By Name(cluster=w24, "Temp (F)"=w32, "FIB Faraday Cup (nA)"=w31, "FIB Specimen I (nA)"=w30, "Beam Dump 1 (nA)"=w29, "Beam Dump 2 (nA)"=w3, "Milling I (nA)"=w2, "SEM Specimen I (nA)"=w28, "Milling Z voltage (V)"=w27, "Focus Index"=w26, "FIB slice #"=w25) -> (w23:T5)
      n52 = Close File(refnum=w17, error in=w16) -> ()  [unwired: 2 out]
      n53 = Index Array(array=w155) -> (element #1=w156:sgl, element #2=w154:sgl, element #3=w157:sgl, element #4=w158:sgl)  [unwired: 4 in]
      n54 = Unbundle By Name(w52) -> ("SEM parameters"=w58:T6)
      n55 = Bundle By Name(cluster=w58, "Detector A"=w121, "Detector B"=w122, "Magnification"=w125, "Pixel size"=w126, "Working distance"=w128, "EHT"=w127, "Aperture"=w131, "High current mode"=w132, "Probe current"=w137, "Scan rotation"=w138, "Chamber vac"=w139, "Gun vac"=w140, "Beam shift X"=w141, "Beam shift Y"=w143, "Stig X"=w144, "Stig Y"=w145, "Alignment X"=w146, "Alignment Y"=w147, "Stage X"=w148, "Stage Y"=w149, "Stage Z"=w150, "Stage T"=w151, "Stage R"=w152, "Stage M"=w153, "Brightness A"=w156, "Contrast A"=w154, "Brightness B"=w157, "Contrast B"=w158) -> (w53:T6)
      n56 = Bundle By Name(cluster=w52, "SEM parameters"=w53, "Other detectors"=w50, "FIB parameters"=w49, "Data Logging"=w23, "Decimating factor"=w15) -> (→"Ouputs":T1)
    }
    frame True {
      n57 = Unbundle By Name("Inputs") -> ("AI sampling time increment"=w262:dbl, "8-bit"=w216:bool, "AI scaling coefficients"=w217:sgl[][], "AI channels"=w270:T7, "Resolution and scan"=w269:T8, "Decimating factor"=w237:u16, "Notes"=w268:string, "Other detectors"=w263:T3, "SEM parameters"=w267:T6, "FIB parameters"=w266:T4, "Milling para"=w265:T9, "Machine ID"=w264:string, "Data Logging"=w261:T5)
      n58 = Unbundle By Name(w261) -> ("Temp (F)"=w260:sgl, "FIB Faraday Cup (nA)"=w259:sgl, "FIB Specimen I (nA)"=w258:sgl, "Beam Dump 1 (nA)"=w257:sgl, "Beam Dump 2 (nA)"=w206:sgl, "Milling I (nA)"=w205:sgl, "SEM Specimen I (nA)"=w256:sgl, "Milling Z voltage (V)"=w255:sgl, "Focus Index"=w254:sgl, "FIB slice #"=w238:u32)
      n59 = Unbundle By Name(w270) -> ("AI 1"=w350:bool, "AI 2"=w349:bool, "AI 3"=w346:bool, "AI 4"=w345:bool)
      n60 = Unbundle By Name(w269) -> ("X resolution"=w517:u32, "Z resolution"=w516:u32, "AI oversampling"=w515:u16, "Scan speed"=w514:u8, "Actual AO rate"=w425:dbl, "Frame line rampdown ratio"=w424:dbl, "X min (V)"=w423:dbl, "X max (V)"=w422:dbl, "Det min (V)"=w342:dbl, "Det max (V)"=w341:dbl)
      n61 = Unbundle By Name(w267) -> ("Detector A"=w431:string, "Detector B"=w430:string, "Magnification"=w388:sgl, "Pixel size"=w387:sgl, "Working distance"=w386:sgl, "EHT"=w385:sgl, "Aperture"=w440:u8, "High current mode"=w439:u8, "Probe current"=w397:sgl, "Scan rotation"=w396:sgl, "Chamber vac"=w395:sgl, "Gun vac"=w394:sgl, "Beam shift X"=w419:sgl, "Beam shift Y"=w418:sgl, "Stig X"=w378:sgl, "Stig Y"=w377:sgl, "Alignment X"=w376:sgl, "Alignment Y"=w375:sgl, "Stage X"=w373:sgl, "Stage Y"=w372:sgl, "Stage Z"=w371:sgl, "Stage T"=w370:sgl, "Stage R"=w369:sgl, "Stage M"=w368:sgl, "Brightness A"=w429:sgl, "Contrast A"=w428:sgl, "Brightness B"=w426:sgl, "Contrast B"=w427:sgl)
      n62 = Unbundle By Name(w265) -> ("X resolution"=w327:u32, "Z resolution"=w326:u32, "X size (um)"=w324:sgl, "Z size (um)"=w323:sgl, "UL-Ang"=w322:sgl, "UR-Ang"=w321:sgl, "Line milling time (s)"=w320:sgl, "Lines auto pause"=w308:u16, "FIB FOV (um)"=w305:sgl, "FIB PID on"=w287:bool, "FIB PID measured"=w227:u8, "FIB PID target"=w304:sgl, "FIB PID target slope"=w303:sgl, "FIB PID P"=w302:sgl, "FIB PID I"=w301:sgl, "FIB PID D"=w300:sgl)
      n63 = Unbundle By Name(w266) -> ("FIB mode"=w443:u8, "FIB focus"=w442:sgl, "FIB probe current"=w441:u8, "FIB emission current"=w365:sgl, "FIB rotation"=w364:sgl, "FIB aperture X"=w363:sgl, "FIB aperture Y"=w362:sgl, "FIB stig X"=w361:sgl, "FIB stig Y"=w360:sgl, "FIB beam shift X"=w359:sgl, "FIB beam shift Y"=w358:sgl)
      n64 = Set File Position(offset (in bytes) (0)=0 ("pos offset (0)"), refnum="refnum", from (0:start)=enum16{"start", "end", "current"}."start" ("pos mode (0:2)"), error in="error in") -> (refnum out=w565:refnum<file>, error out=w564:errorcluster)
      n65 = Write to Binary File(file (use dialog)=w565, data=u32 3555587570, error in=w564, 5:FALSE ("prepend array or string size? (T)")) -> (refnum out=w604:refnum<file>, error out=w601:errorcluster)  [unwired: 3 out]
      n66 = Build Array(w260, w259, w258, w257, w256, w255, w254) -> (w239:sgl[])
      n67 = Build Array(w388, w387, w386, w385) -> (w384:sgl[])
      n68 = Build Array(w440, w439) -> (w381:u8[])
      n69 = Build Array(w397, w396, w395, w394) -> (w380:sgl[])
      n70 = Build Array(w419, w418, w378, w377, w376, w375, w373, w372, w371, w370, w369, w368) -> (w379:sgl[])
      n71 = Build Array(w429, w428, w426, w427) -> (w374:sgl[])
      n72 = Set File Position(offset (in bytes) (0)=4 ("pos offset (0)"), refnum=w604, from (0:start)=enum16{"start", "end", "current"}."start" ("pos mode (0:2)"), error in=w601) -> (refnum out=w568:refnum<file>, error out=w567:errorcluster)
      n73 = Build Array(w365, w364, w363, w362, w361, w360, w359, w358) -> (w357:sgl[])
      n74 = Build Array(w327, w326) -> (w325:u32[])
      n75 = Build Array(w324, w323, w322, w321, w320, w305) -> (w314:sgl[])
      n76 = Build Array(w304, w303, w302, w301, w300) -> (w284:sgl[])
      n77 = Build Array(w350, w349, w346, w345) -> (w389:bool[])
      n78 = Build Array(w206, w205) -> (w204:sgl[])
      n79 = Build Array(w425, w424, w423, w422, w342, w341) -> (w421:dbl[])
      n80 = Write to Binary File(file (use dialog)=w568, data=u16 8, error in=w567, 5:FALSE ("prepend array or string size? (T)")) -> (refnum out=w595:refnum<file>, error out=w594:errorcluster)  [unwired: 3 out]
      n81 = Set File Position(offset (in bytes) (0)=6 ("pos offset (0)"), refnum=w595, from (0:start)=enum16{"start", "end", "current"}."start" ("pos mode (0:2)"), error in=w594) -> (refnum out=w571:refnum<file>, error out=w570:errorcluster)
      n82 = To Unsigned Word Integer(number=w515) -> (unsigned 16bit integer=w420:u16)
      n83 = To Single Precision Float(number=w421) -> (single precision float=w340:sgl[])
      n84 = Write to Binary File(file (use dialog)=w571, data=u16 1, error in=w570, 5:FALSE ("prepend array or string size? (T)")) -> (refnum out=w276:refnum<file>, error out=w275:errorcluster)  [unwired: 3 out]
      n85 = Unbundle By Name(w263) -> ("Detector C name"=w401:string, "Detector D name"=w400:string)
      n86 = shared-variable ".\\Zeiss Library.lvlib\\SW date"() -> (w272:string)  [unwired: 1 in, 1 out]
      "SW date" <- w272
      n87 = Set File Position(offset (in bytes) (0)=8 ("pos offset (0)"), refnum=w276, from (0:start)=enum16{"start", "end", "current"}."start" ("pos mode (0:2)"), error in=w275) -> (refnum out=w279:refnum<file>, error out=w280:errorcluster)
      n88 = Write to Binary File(file (use dialog)=w279, data=w272, error in=w280, 5:FALSE ("prepend array or string size? (T)")) -> (refnum out=w274:refnum<file>, error out=w273:errorcluster)  [unwired: 3 out]
      n89 = Set File Position(offset (in bytes) (0)=24 ("pos offset (0)"), refnum=w274, from (0:start)=enum16{"start", "end", "current"}."start" ("pos mode (0:2)"), error in=w273) -> (refnum out=w574:refnum<file>, error out=w573:errorcluster)
      n90 = Write to Binary File(file (use dialog)=w574, data=w262, error in=w573, 5:FALSE ("prepend array or string size? (T)")) -> (refnum out=w589:refnum<file>, error out=w588:errorcluster)  [unwired: 3 out]
      n91 = Boolean To (0,1)(Boolean=w350) -> (0, 1=w353:i16)
      n92 = Boolean To (0,1)(Boolean=w349) -> (0, 1=w352:i16)
      n93 = Boolean To (0,1)(Boolean=w346) -> (0, 1=w348:i16)
      n94 = Boolean To (0,1)(Boolean=w345) -> (0, 1=w347:i16)
      n95 = Compound Arithmetic op=ADD(w353, w352, w348, w347) -> (w351:i16)
      n96 = To Unsigned Byte Integer(number=w351) -> (unsigned 8bit integer=w581:u8)
      n97 = Set File Position(offset (in bytes) (0)=32 ("pos offset (0)"), refnum=w589, from (0:start)=enum16{"start", "end", "current"}."start" ("pos mode (0:2)"), error in=w588) -> (refnum out=w577:refnum<file>, error out=w576:errorcluster)
      n98 = Write to Binary File(file (use dialog)=w577, data=w581, error in=w576, 5:FALSE ("prepend array or string size? (T)")) -> (refnum out=w585:refnum<file>, error out=w584:errorcluster)  [unwired: 3 out]
      n99 = Set File Position(offset (in bytes) (0)=33 ("pos offset (0)"), refnum=w585, from (0:start)=enum16{"start", "end", "current"}."start" ("pos mode (0:2)"), error in=w584) -> (refnum out=w580:refnum<file>, error out=w579:errorcluster)
      n100 = Write to Binary File(file (use dialog)=w580, data=w216, error in=w579, 5:FALSE ("prepend array or string size? (T)")) -> (refnum out=w219:refnum<file>, error out=w221:errorcluster)  [unwired: 3 out]
      n101 = Set File Position(offset (in bytes) (0)=36 ("pos offset (0)"), refnum=w219, from (0:start)=enum16{"start", "end", "current"}."start" ("pos mode (0:2)"), error in=w221) -> (refnum out=w224:refnum<file>, error out=w225:errorcluster)
      n102 = Write to Binary File(file (use dialog)=w224, data=w217, error in=w225, 5:FALSE ("prepend array or string size? (T)")) -> (refnum out=w218:refnum<file>, error out=w220:errorcluster)  [unwired: 3 out]
      n103 = Set File Position(offset (in bytes) (0)=100 ("pos offset (0)"), refnum=w218, from (0:start)=enum16{"start", "end", "current"}."start" ("pos mode (0:2)"), error in=w220) -> (refnum out=w556:refnum<file>, error out=w557:errorcluster)
      n104 = Write to Binary File(file (use dialog)=w556, data=w517, error in=w557, 5:FALSE ("prepend array or string size? (T)")) -> (refnum out=w540:refnum<file>, error out=w539:errorcluster)  [unwired: 3 out]
      n105 = Set File Position(offset (in bytes) (0)=104 ("pos offset (0)"), refnum=w540, from (0:start)=enum16{"start", "end", "current"}."start" ("pos mode (0:2)"), error in=w539) -> (refnum out=w549:refnum<file>, error out=w548:errorcluster)
      n106 = Write to Binary File(file (use dialog)=w549, data=w516, error in=w548, 5:FALSE ("prepend array or string size? (T)")) -> (refnum out=w542:refnum<file>, error out=w541:errorcluster)  [unwired: 3 out]
      n107 = Set File Position(offset (in bytes) (0)=108 ("pos offset (0)"), refnum=w542, from (0:start)=enum16{"start", "end", "current"}."start" ("pos mode (0:2)"), error in=w541) -> (refnum out=w546:refnum<file>, error out=w547:errorcluster)
      n108 = Write to Binary File(file (use dialog)=w546, data=w420, error in=w547, 5:FALSE ("prepend array or string size? (T)")) -> (refnum out=w344:refnum<file>, error out=w343:errorcluster)  [unwired: 3 out]
      n109 = Set File Position(offset (in bytes) (0)=111 ("pos offset (0)"), refnum=w344, from (0:start)=enum16{"start", "end", "current"}."start" ("pos mode (0:2)"), error in=w343) -> (refnum out=w535:refnum<file>, error out=w534:errorcluster)
      n110 = Write to Binary File(file (use dialog)=w535, data=w514, error in=w534, 5:FALSE ("prepend array or string size? (T)")) -> (refnum out=w528:refnum<file>, error out=w527:errorcluster)  [unwired: 3 out]
      n111 = Set File Position(offset (in bytes) (0)=112 ("pos offset (0)"), refnum=w528, from (0:start)=enum16{"start", "end", "current"}."start" ("pos mode (0:2)"), error in=w527) -> (refnum out=w532:refnum<file>, error out=w533:errorcluster)
      n112 = Write to Binary File(file (use dialog)=w532, data=w340, error in=w533, 5:FALSE ("prepend array or string size? (T)")) -> (refnum out=w521:refnum<file>, error out=w520:errorcluster)  [unwired: 3 out]
      n113 = Set File Position(offset (in bytes) (0)=136 ("pos offset (0)"), refnum=w521, from (0:start)=enum16{"start", "end", "current"}."start" ("pos mode (0:2)"), error in=w520) -> (refnum out=w525:refnum<file>, error out=w526:errorcluster)
      n114 = Write to Binary File(file (use dialog)=w525, data=w237, error in=w526, 5:FALSE ("prepend array or string size? (T)")) -> (refnum out=w519:refnum<file>, error out=w518:errorcluster)  [unwired: 3 out]
      n115 = Set File Position(offset (in bytes) (0)=151 ("pos offset (0)"), refnum=w519, from (0:start)=enum16{"start", "end", "current"}."start" ("pos mode (0:2)"), error in=w518) -> (refnum out=w505:refnum<file>, error out=w504:errorcluster)
      n116 = Write to Binary File(file (use dialog)=w505, data=w389, error in=w504, 5:FALSE ("prepend array or string size? (T)")) -> (refnum out=w391:refnum<file>, error out=w390:errorcluster)  [unwired: 3 out]
      n117 = Set File Position(offset (in bytes) (0)=180 ("pos offset (0)"), refnum=w391, from (0:start)=enum16{"start", "end", "current"}."start" ("pos mode (0:2)"), error in=w390) -> (refnum out=w510:refnum<file>, error out=w509:errorcluster)
      n118 = Write to Binary File(file (use dialog)=w510, data=w268, error in=w509, 5:FALSE ("prepend array or string size? (T)")) -> (refnum out=w393:refnum<file>, error out=w392:errorcluster)  [unwired: 3 out]
      n119 = Set File Position(offset (in bytes) (0)=380 ("pos offset (0)"), refnum=w393, from (0:start)=enum16{"start", "end", "current"}."start" ("pos mode (0:2)"), error in=w392) -> (refnum out=w482:refnum<file>, error out=w481:errorcluster)
      n120 = Write to Binary File(file (use dialog)=w482, data=w431, error in=w481, 5:FALSE ("prepend array or string size? (T)")) -> (refnum out=w433:refnum<file>, error out=w432:errorcluster)  [unwired: 3 out]
      n121 = Set File Position(offset (in bytes) (0)=390 ("pos offset (0)"), refnum=w433, from (0:start)=enum16{"start", "end", "current"}."start" ("pos mode (0:2)"), error in=w432) -> (refnum out=w436:refnum<file>, error out=w435:errorcluster)
      n122 = Write to Binary File(file (use dialog)=w436, data=w430, error in=w435, 5:FALSE ("prepend array or string size? (T)")) -> (refnum out=w405:refnum<file>, error out=w404:errorcluster)  [unwired: 3 out]
      n123 = Set File Position(offset (in bytes) (0)=410 ("pos offset (0)"), refnum=w405, from (0:start)=enum16{"start", "end", "current"}."start" ("pos mode (0:2)"), error in=w404) -> (refnum out=w414:refnum<file>, error out=w415:errorcluster)
      n124 = Write to Binary File(file (use dialog)=w414, data=w401, error in=w415, 5:FALSE ("prepend array or string size? (T)")) -> (refnum out=w416:refnum<file>, error out=w417:errorcluster)  [unwired: 3 out]
      n125 = Set File Position(offset (in bytes) (0)=430 ("pos offset (0)"), refnum=w416, from (0:start)=enum16{"start", "end", "current"}."start" ("pos mode (0:2)"), error in=w417) -> (refnum out=w407:refnum<file>, error out=w406:errorcluster)
      n126 = Write to Binary File(file (use dialog)=w407, data=w400, error in=w406, 5:FALSE ("prepend array or string size? (T)")) -> (refnum out=w403:refnum<file>, error out=w402:errorcluster)  [unwired: 3 out]
      n127 = Set File Position(offset (in bytes) (0)=460 ("pos offset (0)"), refnum=w403, from (0:start)=enum16{"start", "end", "current"}."start" ("pos mode (0:2)"), error in=w402) -> (refnum out=w485:refnum<file>, error out=w484:errorcluster)
      n128 = Write to Binary File(file (use dialog)=w485, data=w384, error in=w484, 5:FALSE ("prepend array or string size? (T)")) -> (refnum out=w497:refnum<file>, error out=w496:errorcluster)  [unwired: 3 out]
      n129 = Set File Position(offset (in bytes) (0)=480 ("pos offset (0)"), refnum=w497, from (0:start)=enum16{"start", "end", "current"}."start" ("pos mode (0:2)"), error in=w496) -> (refnum out=w488:refnum<file>, error out=w487:errorcluster)
      n130 = Write to Binary File(file (use dialog)=w488, data=w381, error in=w487, 5:FALSE ("prepend array or string size? (T)")) -> (refnum out=w493:refnum<file>, error out=w492:errorcluster)  [unwired: 3 out]
      n131 = Set File Position(offset (in bytes) (0)=490 ("pos offset (0)"), refnum=w493, from (0:start)=enum16{"start", "end", "current"}."start" ("pos mode (0:2)"), error in=w492) -> (refnum out=w491:refnum<file>, error out=w490:errorcluster)
      n132 = Write to Binary File(file (use dialog)=w491, data=w380, error in=w490, 5:FALSE ("prepend array or string size? (T)")) -> (refnum out=w383:refnum<file>, error out=w382:errorcluster)  [unwired: 3 out]
      n133 = Set File Position(offset (in bytes) (0)=510 ("pos offset (0)"), refnum=w383, from (0:start)=enum16{"start", "end", "current"}."start" ("pos mode (0:2)"), error in=w382) -> (refnum out=w478:refnum<file>, error out=w479:errorcluster)
      n134 = Write to Binary File(file (use dialog)=w478, data=w379, error in=w479, 5:FALSE ("prepend array or string size? (T)")) -> (refnum out=w399:refnum<file>, error out=w398:errorcluster)  [unwired: 3 out]
      n135 = Set File Position(offset (in bytes) (0)=560 ("pos offset (0)"), refnum=w399, from (0:start)=enum16{"start", "end", "current"}."start" ("pos mode (0:2)"), error in=w398) -> (refnum out=w560:refnum<file>, error out=w561:errorcluster)
      n136 = Write to Binary File(file (use dialog)=w560, data=w374, error in=w561, 5:FALSE ("prepend array or string size? (T)")) -> (refnum out=w366:refnum<file>, error out=w367:errorcluster)  [unwired: 3 out]
      n137 = Set File Position(offset (in bytes) (0)=600 ("pos offset (0)"), refnum=w366, from (0:start)=enum16{"start", "end", "current"}."start" ("pos mode (0:2)"), error in=w367) -> (refnum out=w472:refnum<file>, error out=w473:errorcluster)
      n138 = Write to Binary File(file (use dialog)=w472, data=w443, error in=w473, 5:FALSE ("prepend array or string size? (T)")) -> (refnum out=w469:refnum<file>, error out=w468:errorcluster)  [unwired: 3 out]
      n139 = Set File Position(offset (in bytes) (0)=604 ("pos offset (0)"), refnum=w469, from (0:start)=enum16{"start", "end", "current"}."start" ("pos mode (0:2)"), error in=w468) -> (refnum out=w446:refnum<file>, error out=w445:errorcluster)
      n140 = Write to Binary File(file (use dialog)=w446, data=w442, error in=w445, 5:FALSE ("prepend array or string size? (T)")) -> (refnum out=w463:refnum<file>, error out=w462:errorcluster)  [unwired: 3 out]
      n141 = Set File Position(offset (in bytes) (0)=608 ("pos offset (0)"), refnum=w463, from (0:start)=enum16{"start", "end", "current"}."start" ("pos mode (0:2)"), error in=w462) -> (refnum out=w449:refnum<file>, error out=w448:errorcluster)
      n142 = Write to Binary File(file (use dialog)=w449, data=w441, error in=w448, 5:FALSE ("prepend array or string size? (T)")) -> (refnum out=w459:refnum<file>, error out=w458:errorcluster)  [unwired: 3 out]
      n143 = Set File Position(offset (in bytes) (0)=620 ("pos offset (0)"), refnum=w459, from (0:start)=enum16{"start", "end", "current"}."start" ("pos mode (0:2)"), error in=w458) -> (refnum out=w452:refnum<file>, error out=w451:errorcluster)
      n144 = Write to Binary File(file (use dialog)=w452, data=w357, error in=w451, 5:FALSE ("prepend array or string size? (T)")) -> (refnum out=w329:refnum<file>, error out=w328:errorcluster)  [unwired: 3 out]
      n145 = Set File Position(offset (in bytes) (0)=652 ("pos offset (0)"), refnum=w329, from (0:start)=enum16{"start", "end", "current"}."start" ("pos mode (0:2)"), error in=w328) -> (refnum out=w332:refnum<file>, error out=w333:errorcluster)
      n146 = Write to Binary File(file (use dialog)=w332, data=w325, error in=w333, 5:FALSE ("prepend array or string size? (T)")) -> (refnum out=w307:refnum<file>, error out=w306:errorcluster)  [unwired: 3 out]
      n147 = Set File Position(offset (in bytes) (0)=660 ("pos offset (0)"), refnum=w307, from (0:start)=enum16{"start", "end", "current"}."start" ("pos mode (0:2)"), error in=w306) -> (refnum out=w317:refnum<file>, error out=w316:errorcluster)
      n148 = Write to Binary File(file (use dialog)=w317, data=w314, error in=w316, 5:FALSE ("prepend array or string size? (T)")) -> (refnum out=w289:refnum<file>, error out=w288:errorcluster)  [unwired: 3 out]
      n149 = Set File Position(offset (in bytes) (0)=684 ("pos offset (0)"), refnum=w289, from (0:start)=enum16{"start", "end", "current"}."start" ("pos mode (0:2)"), error in=w288) -> (refnum out=w311:refnum<file>, error out=w312:errorcluster)
      n150 = Write to Binary File(file (use dialog)=w311, data=w308, error in=w312, 5:FALSE ("prepend array or string size? (T)")) -> (refnum out=w286:refnum<file>, error out=w285:errorcluster)  [unwired: 3 out]
      n151 = Set File Position(offset (in bytes) (0)=686 ("pos offset (0)"), refnum=w286, from (0:start)=enum16{"start", "end", "current"}."start" ("pos mode (0:2)"), error in=w285) -> (refnum out=w292:refnum<file>, error out=w293:errorcluster)
      n152 = Write to Binary File(file (use dialog)=w292, data=w287, error in=w293, 5:FALSE ("prepend array or string size? (T)")) -> (refnum out=w231:refnum<file>, error out=w228:errorcluster)  [unwired: 3 out]
      n153 = Set File Position(offset (in bytes) (0)=689 ("pos offset (0)"), refnum=w231, from (0:start)=enum16{"start", "end", "current"}."start" ("pos mode (0:2)"), error in=w228) -> (refnum out=w234:refnum<file>, error out=w233:errorcluster)
      n154 = Write to Binary File(file (use dialog)=w234, data=w227, error in=w233, 5:FALSE ("prepend array or string size? (T)")) -> (refnum out=w230:refnum<file>, error out=w229:errorcluster)  [unwired: 1 in, 2 out]
      n155 = Set File Position(offset (in bytes) (0)=690 ("pos offset (0)"), refnum=w230, from (0:start)=enum16{"start", "end", "current"}."start" ("pos mode (0:2)"), error in=w229) -> (refnum out=w297:refnum<file>, error out=w296:errorcluster)
      n156 = Write to Binary File(file (use dialog)=w297, data=w284, error in=w296, 5:FALSE ("prepend array or string size? (T)")) -> (refnum out=w283:refnum<file>, error out=w282:errorcluster)  [unwired: 3 out]
      n157 = Set File Position(offset (in bytes) (0)=800 ("pos offset (0)"), refnum=w283, from (0:start)=enum16{"start", "end", "current"}."start" ("pos mode (0:2)"), error in=w282) -> (refnum out=w337:refnum<file>, error out=w338:errorcluster)
      n158 = Write to Binary File(file (use dialog)=w337, data=w264, error in=w338, 5:FALSE ("prepend array or string size? (T)")) -> (refnum out=w241:refnum<file>, error out=w240:errorcluster)  [unwired: 3 out]
      n159 = Set File Position(offset (in bytes) (0)=850 ("pos offset (0)"), refnum=w241, from (0:start)=enum16{"start", "end", "current"}."start" ("pos mode (0:2)"), error in=w240) -> (refnum out=w249:refnum<file>, error out=w250:errorcluster)
      n160 = Write to Binary File(file (use dialog)=w249, data=w239, error in=w250, 5:FALSE ("prepend array or string size? (T)")) -> (refnum out=w252:refnum<file>, error out=w253:errorcluster)  [unwired: 3 out]
      n161 = Set File Position(offset (in bytes) (0)=878 ("pos offset (0)"), refnum=w252, from (0:start)=enum16{"start", "end", "current"}."start" ("pos mode (0:2)"), error in=w253) -> (refnum out=w244:refnum<file>, error out=w243:errorcluster)
      n162 = Write to Binary File(file (use dialog)=w244, data=w238, error in=w243, 5:FALSE ("prepend array or string size? (T)")) -> (refnum out=w210:refnum<file>, error out=w209:errorcluster)  [unwired: 3 out]
      n163 = Set File Position(offset (in bytes) (0)=882 ("pos offset (0)"), refnum=w210, from (0:start)=enum16{"start", "end", "current"}."start" ("pos mode (0:2)"), error in=w209) -> (refnum out=w213:refnum<file>, error out=w214:errorcluster)
      n164 = Write to Binary File(file (use dialog)=w213, data=w204, error in=w214, 5:FALSE ("prepend array or string size? (T)")) -> (refnum out=w208:refnum<file>, error out=w207:errorcluster)  [unwired: 3 out]
      n165 = Set File Position(offset (in bytes) (0)=1023 ("pos offset (0)"), refnum=w208, from (0:start)=enum16{"start", "end", "current"}."start" ("pos mode (0:2)"), error in=w207) -> (refnum out=w455:refnum<file>, error out=w454:errorcluster)
      n166 = Write to Binary File(file (use dialog)=w455, data=i8 0, error in=w454, 5:FALSE ("prepend array or string size? (T)")) -> (refnum out=→"dup refnum":refnum<file>, error out=→"error out":errorcluster)  [unwired: 3 out]
    }
  }
